vi "Loop times Counter.vi"(11 "times":i32[](array[numeric])) -> (1 "Recording?":bool, 2 "Save file?":bool, 3 "Display value?":bool)   [LabVIEW 2018]
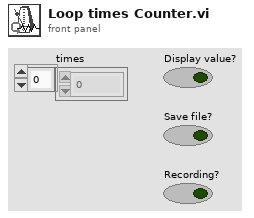
[diagram p1: front panel]
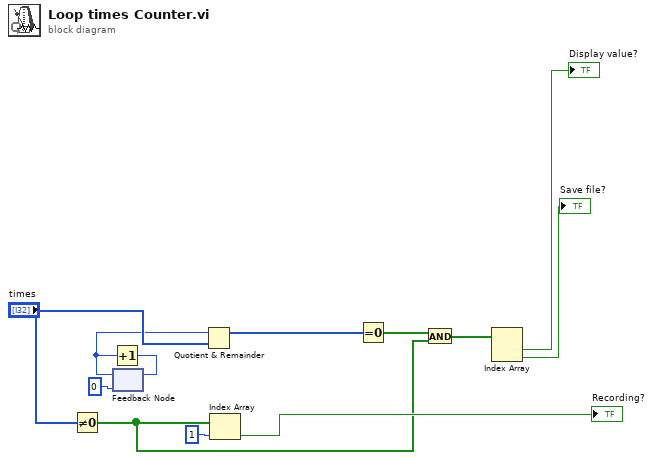
[diagram p0: block diagram]
diagram:
  n1 = Not Equal To 0?(x="times") -> (x != 0?=w10:bool[])
  n2 = feedback #1(0) -> (w3:i32)
  n3 = Increment(x=w3) -> (x+1=w1:i32)
  n4 = feedback-in #1(w1) -> ()
  n5 = Quotient & Remainder(x=w3, y="times") -> (x-y*floor(x/y)=w4:i32[])  [unwired: 1 out]
  n6 = Index Array(array=w10, index=1) -> (element=→"Recording?":bool)
  n7 = Equal To 0?(x=w4) -> (x = 0?=w8:bool[])
  n8 = And(x=w8, y=w10) -> (x .and. y?=w9:bool[])
  n9 = Index Array(array=w9) -> (element #1=→"Display value?":bool, element #2=→"Save file?":bool)  [unwired: 2 in]
